vi "Panel Launcher Demo.vi"() -> ()   [LabVIEW 2012]
doc: "This VI demonstrates how to implement the Panel Launcher XControl example. The Panel Launcher is a custom XControl button that you can configure to launch a variety of tasks interactively."
uses:
  Panel Launcher XControl/PanelWizard.xctl
panel:
  in  "Run User VI":bool(xcontrol)
  out "String":string="Instructions:\n\nThe buttons below are instances of custom XControl that extends the basic LabVIEW boolean control.\nOpen the project PanelWizard.lvproj in the examples folder to see how the XControl was constructed.\n\nThe buttons below implement a special right-click menu feature that allows you to configure actions to occur when the buttons are pressed.  Right-click the buttons and choose \"Configure Panel Wizard ...\" to configure the buttons."
  in  "Run Command Line":bool(xcontrol)
  in  "Launch System Manager":bool(xcontrol)
  in  "Launch HDV":bool(xcontrol)
  # "DSC Module Example Program\nPanel Launcher XControl"
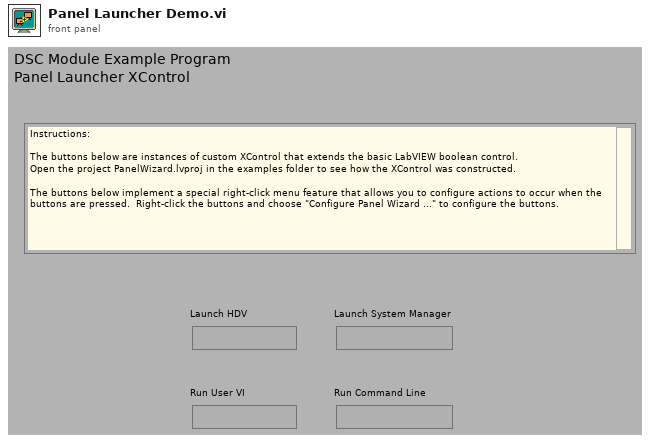
[diagram p1: front panel]
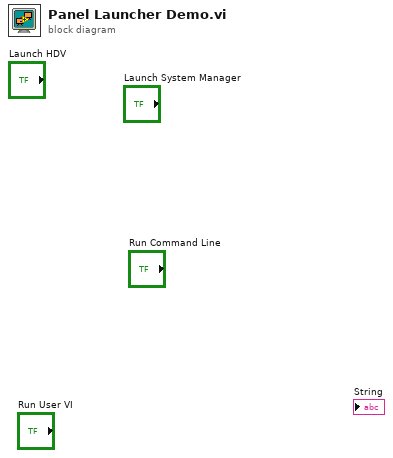
[diagram p0: block diagram]
diagram:
